vi "KNN clasification.vi"() -> ()   [LabVIEW 2014]
uses:
  <vilib>/Utility/file.llb/Write To Spreadsheet File (string).vi
panel:
  out "results":string[][](array[string])
  in  "cluster centers (original) 2":string[](array[string])=["1 0 -1 1 -1 0 -4 1 -4 0 1", "2 0 -1 2 -1 0 -2 2 -2 0 2", "3 0 -3 3 -3 0 -2 3 -2 0 3", "4 0 -3 4 -3 0 -4 4 -4 0 4", "-1 1 -4 0 -4 4 -3 4 -4 0 -4 1 -1", "-1 2 -2 0 -2 3 -3 3 -2 0 -2 2 -1", "-4 1 -1 0 -1 2 -2 2 -1 0 -1 1 -4", "-4 4 -3 0 -3 3 -2 3 -3 0 -3 4 -4", "0 -4 1 -1 0 -3 3 -2 3 -3 0 -1 1 -4 0", "0 -4 4 -3 0 -1 2 -2 2 -1 0 -3 4 -4 0"]
  in  "cluster centers 2 centers for diagonals - short - original clusters":string[](array[string])=["1 0 -1 1 -1 0 -4 1 -4 0 1", "2 0 -1 2 -1 0 -2 2 -2 0 2", "3 0 -3 3 -3 0 -2 3 -2 0 3", "4 0 -3 4 -3 0 -4 4 -4 0 4", "-1 1 -4 0 -4 4 -3 4 -4 0 -4 1 -1", "-1 2 -2 0 -2 3 -3 3 -2 0 -2 2 -1", "-4 1 -1 0 -1 2 -2 2 -1 0 -1 1 -4", "-4 4 -3 0 -3 3 -2 3 -3 0 -3 4 -4", "0 1 -1 0 -3 3 0 3 -3 0 -1 1 0", "0 1 -4 0 -2 3 0 3 -2 0 -4 1 0", "0 4 -3 0 -1 2 0 2 -1 0 -3 4 0", "0 4 -4 0 -2 2 0 2 -2 0 -4 4 0"]
  in  "cluster centers (original)":string[](array[string])=["1 0 -1 1 -1 0 -4 1 -4 0 1", "2 0 -1 2 -1 0 -2 2 -2 0 2", "3 0 -3 3 -3 0 -2 3 -2 0 3", "4 0 -3 4 -3 0 -4 4 -4 0 4", "-1 1 -4 0 -4 4 -3 4 -4 0 -4 1 -1", "-1 2 -2 0 -2 3 -3 3 -2 0 -2 2 -1", "-4 1 -1 0 -1 2 -2 2 -1 0 -1 1 -4", "-4 4 -3 0 -3 3 -2 3 -3 0 -3 4 -4", "0 -4 1 -1 0 -3 3 -2 3 -3 0 -1 1 -4 0", "0 -4 4 -3 0 -1 2 -2 2 -1 0 -3 4 -4 0"]
  out "data to save":string[][](array[string])
  out "position only":string[][](array[string])
  out "non directional transition":string[][](array[string])
  in  "ALL data in checked":string[][](array[string])=array2194x3[6582 elements]
  in  "from CSS validation cluster centers 2 centers for diagonals - long - original clusters 3":string[](array[string])=["1 0 -1 1 -1 0 -4 1 -4 0 1 0 -1 1 -1 0 -4 1 -4 0 1 0 -1 1 -1 0 -4 1 -4 0 1", "2 0 -1 2 -1 0 -2 2 -2 0 2 0 -1 2 -1 0 -2 2 -2 0 2 0 -1 2 -1 0 -2 2 -2 0 2", "3 0 -3 3 -3 0 -2 3 -2 0 3 0 -3 3 -3 0 -2 3 -2 0 3 0 -3 3 -3 0 -2 3 -2 0 3", "4 0 -3 4 -3 0 -4 4 -4 0 4 0 -3 4 -3 0 -4 4 -4 0 4 0 -3 4 -3 0 -4 4 -4 0 4", "-1 1 -4 0 -4 4 -3 4 -4 0 -4 1 -1 1 -4 0 -4 4 -3 4 -4 0 -4 1 -1 1 -4 0 -4 4 -3 4 -4 0 -4 1 -1", "-1 2 -2 0 -2 3 -3 3 -2 0 -2 2 -1 2 -2 0 -2 3 -3 3 -2 0 -2 2 -1 2 -2 0 -2 3 -3 3 -2 0 -2 2 -1", "-4 1 -1 0 -1 2 -2 2 -1 0 -1 1 -4 1 -1 0 -1 2 -2 2 -1 0 -1 1 -4 1 -1 0 -1 2 -2 2 -1 0 -1 1 -4", "-4 4 -3 0 -3 3 -2 3 -3 0 -3 4 -4 4 -3 0 -3 3 -2 3 -3 0 -3 4 -4 4 -3 0 -3 3 -2 3 -3 0 -3 4 -4", "0 1 -1 0 -3 3 0 3 -3 0 -1 1 0 1 -1 0 -3 3 0 3 -3 0 -1 1 0 1 -1 0 -3 3 0 3 -3 0 -1 1 0 ", "0 1 -4 0 -2 3 0 3 -2 0 -4 1 0 1 -4 0 -2 3 0 3 -2 0 -4 1 0 1 -4 0 -2 3 0 3 -2 0 -4 1 0", "0 4 -3 0 -1 2 0 2 -1 0 -3 4 0 4 -3 0 -1 2 0 2 -1 0 -3 4 0 4 -3 0 -1 2 0 2 -1 0 -3 4 0", "0 4 -4 0 -2 2 0 2 -2 0 -4 4 0 4 -4 0 -2 2 0 2 -2 0 -4 4 0 4 -4 0 -2 2 0 2 -2 0 -4 4 0"]
  out "output 2":string[][](array[string])
  in  "K":i32
  in  "cluster centers 2 centers for diagonals - short clusters  with zero side clusters 3 (mod)":string[](array[string])=["0 1 0 -1 1 0 1 -1 0 -4 1 0 1 -4 0", "0 2 0 -1 2 0 2 -1 0 -2 2 0 2 -2 0", "0 3 0 -3 3 0 3 -3 0 -2 3 0 3 -2 0", "0 4 0 -3 4 0 4 -3 0 -4 4 0 4 -4 0", "0 1 0 1 -4 0 -4 4 0 4 0 4 0 4 -4 0 -4 1 0 1 0", "0 2 0 2 -2 0 -2 3 0 3 0 3 0 3 -2 0 -2 2 0 2 0", "0 1 0 1 -1 0 -1 2 0 2 0 2 0 2 -1 0 -1 1 0 1 0", "0 4 0 4 -3 0 -3 3 0 3 0 3 0 3 -3 0 -3 4 0 4 0", "0 1 -1 0 -3 3 0 3 -3 0 -1 1 0 1 -1 0 -3 3 0 3 -3 0 -1 1 0", "0 1 -4 0 -2 3 0 3 -2 0 -4 1 0 1 -4 0 -2 3 0 3 -2 0 -4 1 0", "0 4 -3 0 -1 2 0 2 -1 0 -3 4 0 4 -3 0 -1 2 0 2 -1 0 -3 4 0", "0 4 -4 0 -2 2 0 2 -2 0 -4 4 0 4 -4 0 -2 2 0 2 -2 0 -4 4 0"]
  in  "cluster centers 2 centers for diagonals - short clusters  with zero side clusters 2":string[](array[string])=["0 1 0 -1 1 0 1 -1 0 -4 1 0 1 -4 0", "0 2 0 -1 2 0 2 -1 0 -2 2 0 2 -2 0", "0 3 0 -3 3 0 3 -3 0 -2 3 0 3 -2 0", "0 4 0 -3 4 0 4 -3 0 -4 4 0 4 -4 0", "0 -1 1 0 1 -4 0 -4 4 0 4 -3 0 -3 4 0 4 -4 0 -4 1 0 1 -1 0", "0 -1 2 0 2 -2 0 -2 3 0 3 -3 0 -3 3 0 3 -2 0 -2 2 0 2 -1 0", "0 -4 1 0 1 -1 0 -1 2 0 2 -2 0 -2 2 0 2 -1 0 -1 1 0 1 -4 0", "0 -4 4 0 4 -3 0 -3 3 0 3 -2 0 -2 3 0 3 -3 0 -3 4 0 4 -4 0", "0 1 -1 0 -3 3 0 3 -3 0 -1 1 0 1 -1 0 -3 3 0 3 -3 0 -1 1 0", "0 1 -4 0 -2 3 0 3 -2 0 -4 1 0 1 -4 0 -2 3 0 3 -2 0 -4 1 0", "0 4 -3 0 -1 2 0 2 -1 0 -3 4 0 4 -3 0 -1 2 0 2 -1 0 -3 4 0", "0 4 -4 0 -2 2 0 2 -2 0 -4 4 0 4 -4 0 -2 2 0 2 -2 0 -4 4 0"]
  in  "cluster centers 2 centers for diagonals - long clusters  with zero side clusters":string[](array[string])=["0 1 0 -1 1 0 1 -1 0 -4 1 0 1 -4 0 1 0 -1 1 0 1 -1 0 -4 1 0 1 -4 0", "0 2 0 -1 2 0 2 -1 0 -2 2 0 2 -2 0 2 0 -1 2 0 2 -1 0 -2 2 0 2 -2 0", "0 3 0 -3 3 0 3 -3 0 -2 3 0 3 -2 0 3 0 -3 3 0 3 -3 0 -2 3 0 3 -2 0", "0 4 0 -3 4 0 4 -3 0 -4 4 0 4 -4 0 4 0 -3 4 0 4 -3 0 -4 4 0 4 -4 0", "0 -1 1 -4 0 -4 4 -3 0 -3 4 -4 0 -4 1 -1 0 -1 1 -4 0 -4 4 -3 0 -3 4 -4 0 -4 1 -1 0", "0 -1 2 -2 0 -2 3 -3 0 -3 3 -2 0 -2 2 -1 0 -1 2 -2 0 -2 3 -3 0 -3 3 -2 0 -2 2 -1 0", "0 -4 1 -1 0 -1 2 -2 0 -2 2 -1 0 -1 1 -4 0 -4 1 -1 0 -1 2 -2 0 -2 2 -1 0 -1 1 -4 0", "0 -4 4 -3 0 -3 3 -2 0 -2 3 -3 0 -3 4 -4 0 -4 4 -3 0 -3 3 -2 0 -2 3 -3 0 -3 4 -4 0", "0 1 -1 0 -3 3 0 3 -3 0 -1 1 0 1 -1 0 -3 3 0 3 -3 0 -1 1 0", "0 1 -4 0 -2 3 0 3 -2 0 -4 1 0 1 -4 0 -2 3 0 3 -2 0 -4 1 0", "0 4 -3 0 -1 2 0 2 -1 0 -3 4 0 4 -3 0 -1 2 0 2 -1 0 -3 4 0", "0 4 -4 0 -2 2 0 2 -2 0 -4 4 0 4 -4 0 -2 2 0 2 -2 0 -4 4 0", ""]
  in  "cluster centers 2 long":string[](array[string])=["0 1 0 -1 1 0 1 -1 0 -4 1 0 1 -4 0 1 0 -1 1 0 1 -1 0 -4 1 0 1 -4 0", "0 2 0 -1 2 0 2 -1 0 -2 2 0 2 -2 0 2 0 -1 2 0 2 -1 0 -2 2 0 2 -2 0", "0 3 0 -3 3 0 3 -3 0 -2 3 0 3 -2 0 3 0 -3 3 0 3 -3 0 -2 3 0 3 -2 0", "0 4 0 -3 4 0 4 -3 0 -4 4 0 4 -4 0 4 0 -3 4 0 4 -3 0 -4 4 0 4 -4 0", "0 -1 1 -4 0 -4 4 -3 4 -4 0 -4 1 -1 0 -1 1 -4 0 -4 4 -3 4 -4 0 -4 1 -1 0", "0 -1 2 -2 0 -2 3 -3 3 -2 0 -2 2 -1 0 -1 2 -2 0 -2 3 -3 3 -2 0 -2 2 -1 0", "0 -4 1 -1 0 -1 2 -2 2 -1 0 -1 1 -4 0 -4 1 -1 0 -1 2 -2 2 -1 0 -1 1 -4 0", "0 -4 4 -3 0 -3 3 -2 3 -3 0 -3 4 -4 0 -4 4 -3 0 -3 3 -2 3 -3 0 -3 4 -4 0", "0 -4 1 -1 0 -3 3 -2 3 -3 0 -1 1 -4 0 -4 1 -1 0 -3 3 -2 3 -3 0 -1 1 -4 0", "0 -4 4 -3 0 -1 2 -2 2 -1 0 -3 4 -4 0 -4 4 -3 0 -1 2 -2 2 -1 0 -3 4 -4 0"]
  out "directional transitions":string[][](array[string])
  out "Weighted arrays for movement patterns":dbl[][][](array[numeric])
  out "Weighted arrays of cluster centers":dbl[][][](array[numeric])
  in  "Cluster centers":string[](array[string])=["1 0 1 0 1 0 1 0", "2 0 2 0 2 0 2 0", "3 0 3 0 3 0 3 0", "4 0 4 0 4 0 4 0", "1 0 4 0 1 0 4 0", "2 0 3 0 2 0 3 0", "1 0 2 0 1 0 2 0", "3 0 4 0 3 0 4 0", "1 0 3 0 1 0 3 0", "2 0 4 0 2 0 4 0"]
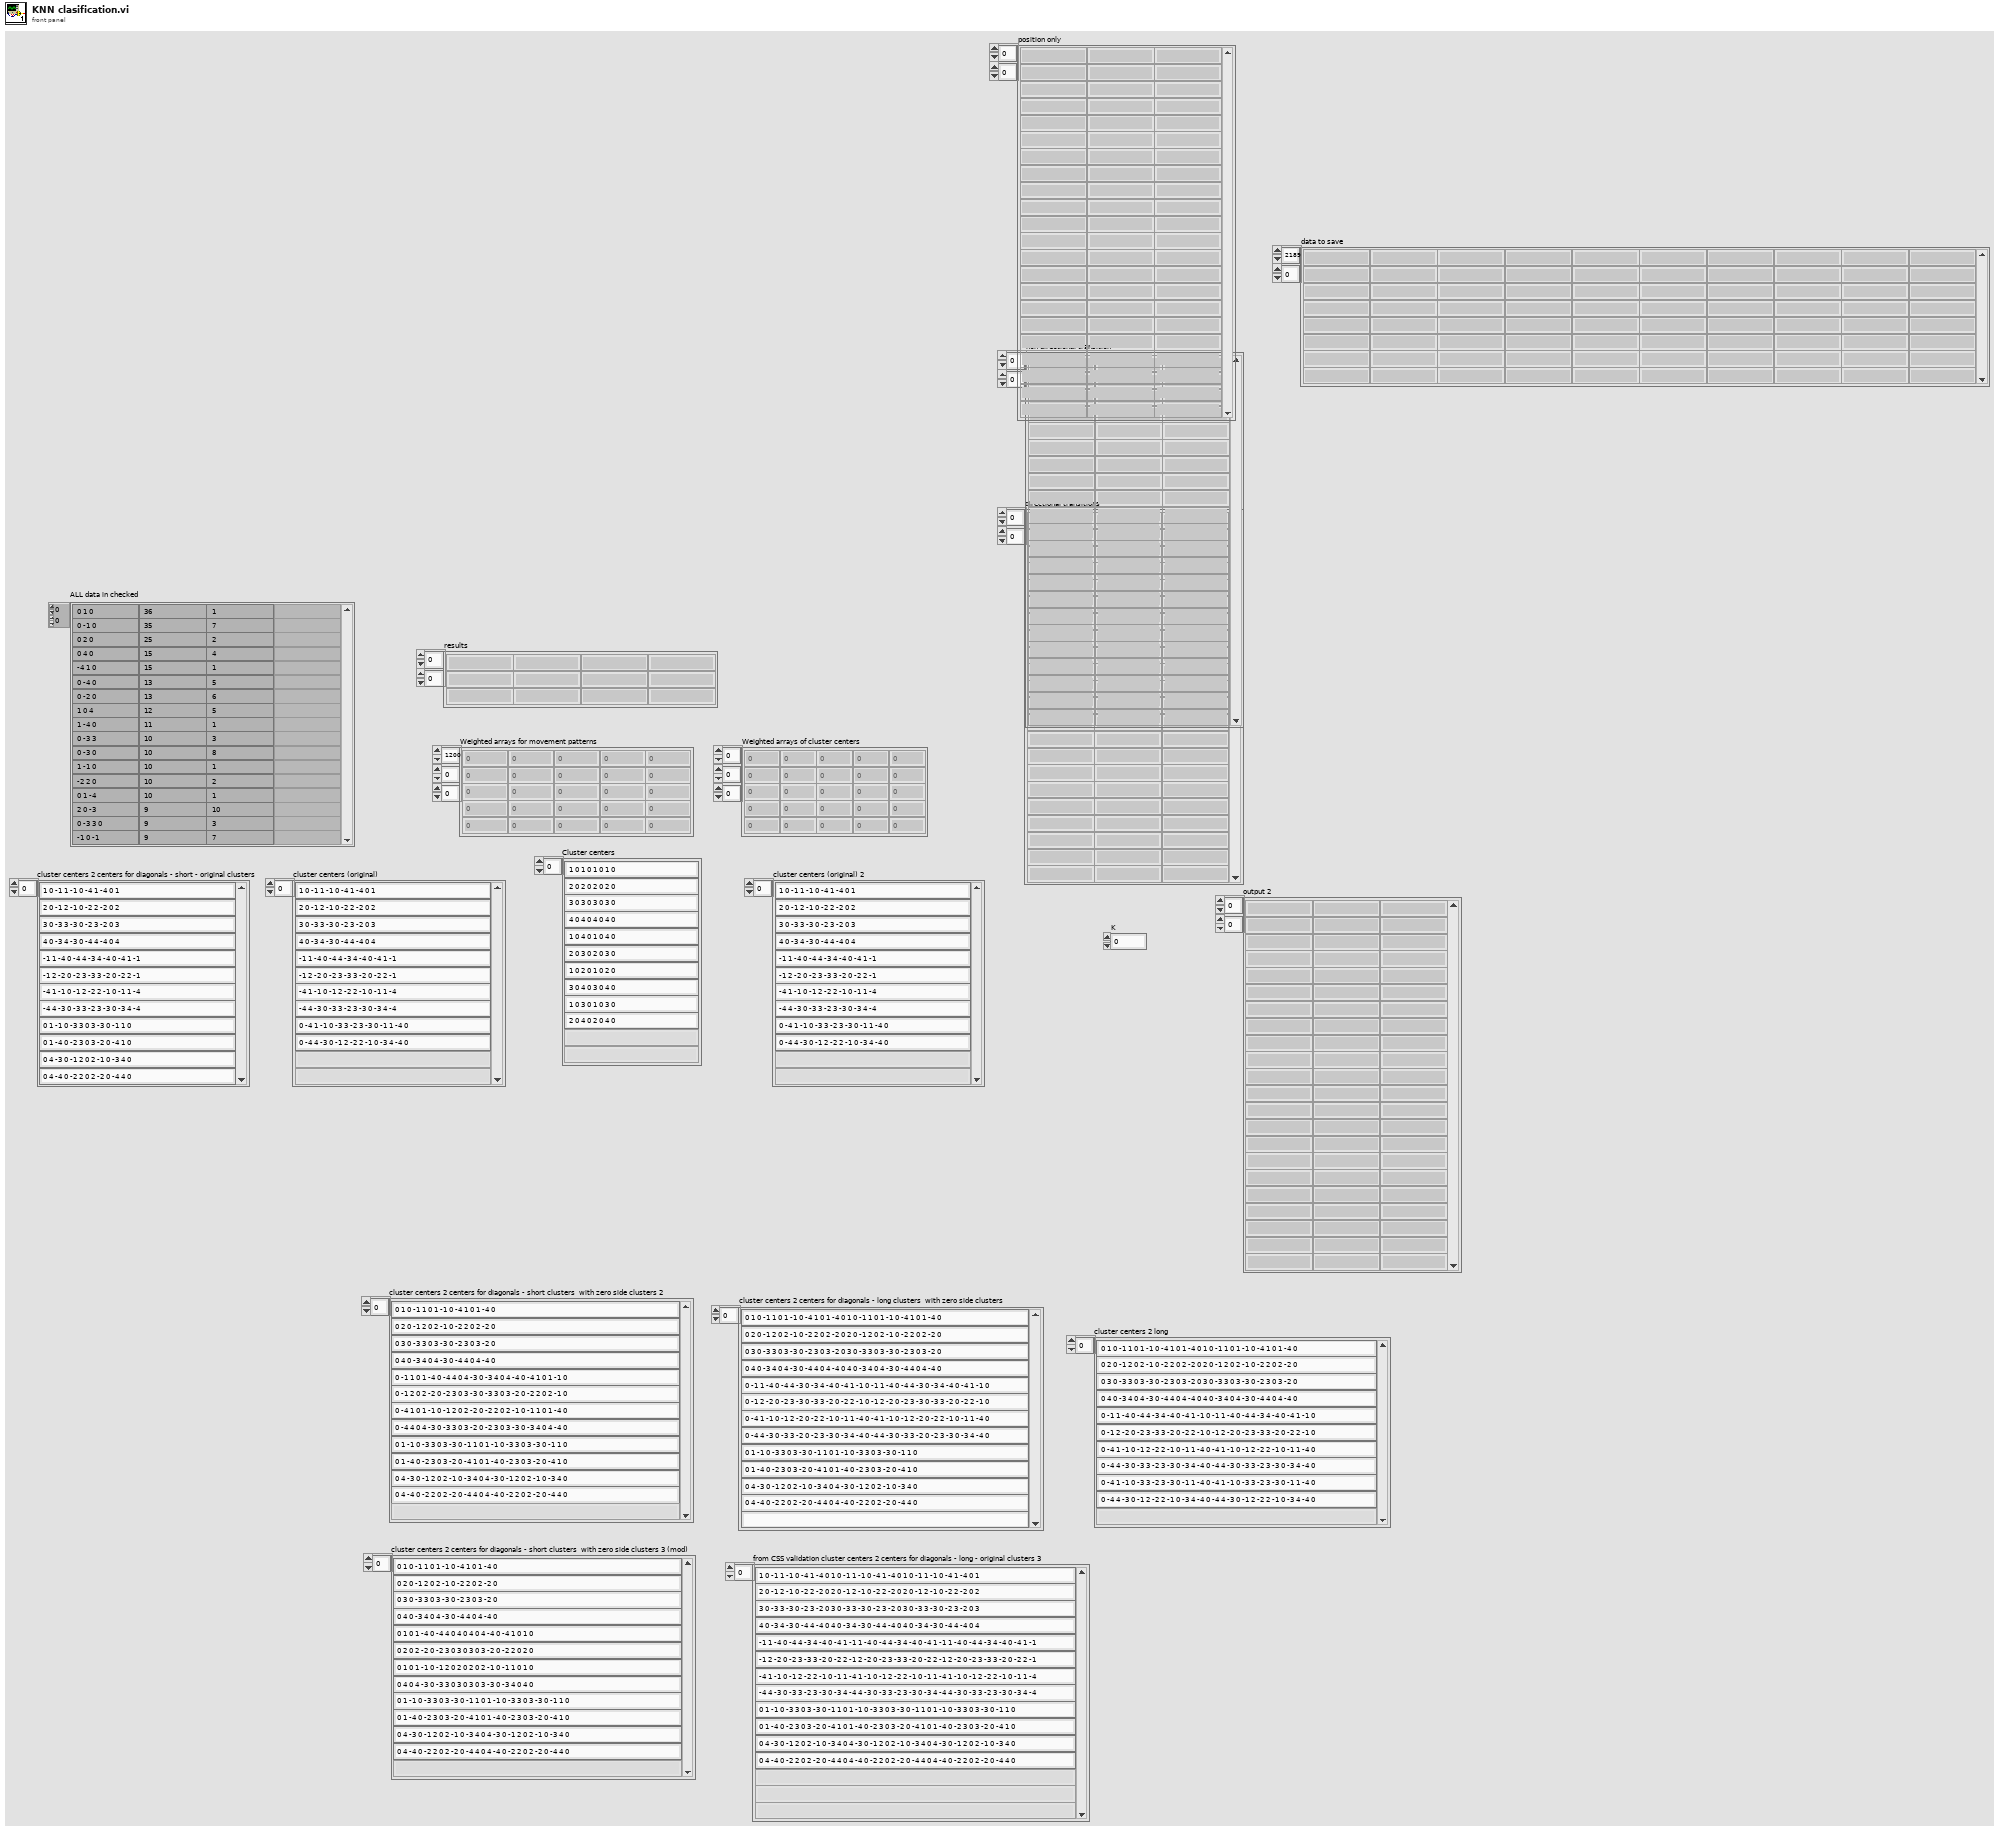
[diagram p1: front panel]
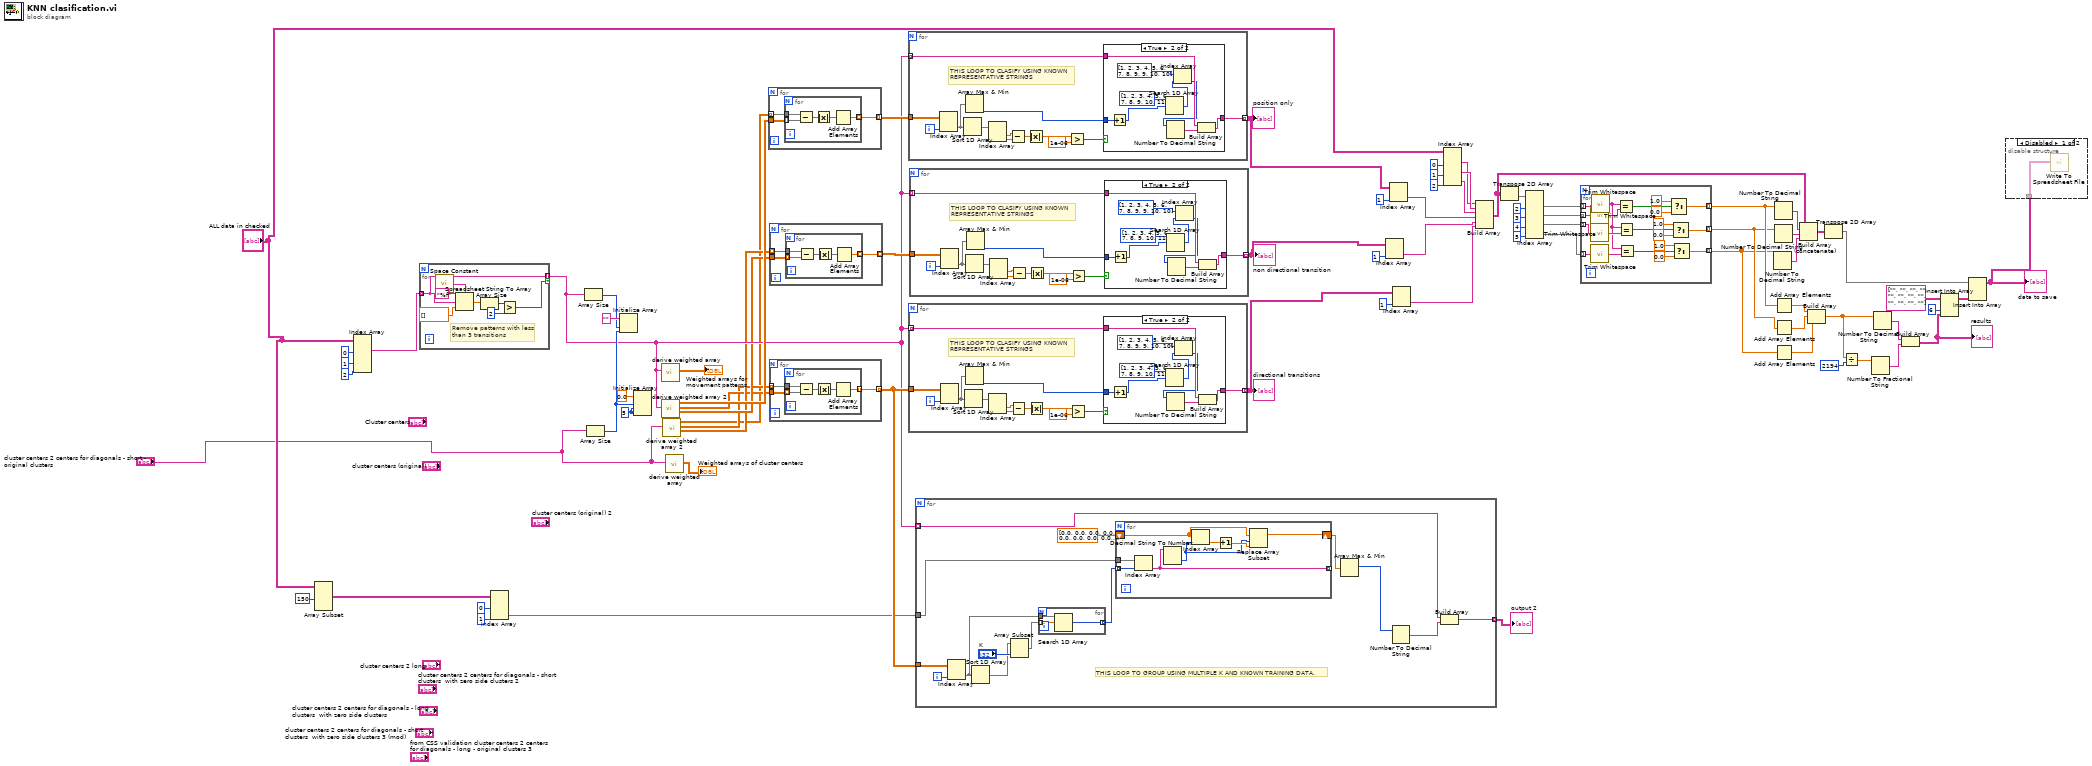
[diagram p0: block diagram]
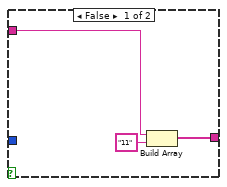
[diagram p3: hidden frame]
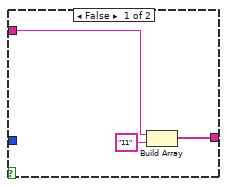
[diagram p4: hidden frame]
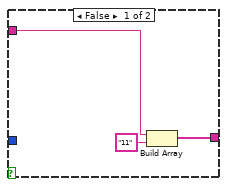
[diagram p5: hidden frame]
diagram:
  w72 = 5 ("dimension size")
  n1 = Array Subset(array="ALL data in checked", length (row)=150 ("length")) -> (w61:string[][])  [unwired: 3 in]
  n2 = Index Array(array="ALL data in checked", index (col) #1=0 ("disabled index (col)"), index (col) #2=1 ("index (col)"), index (col) #3=2 ("index (col)")) -> (element #1=w60:string[])  [unwired: 3 in, 2 out]
  n3 = for {
    tunnel: w60 -> [w77] mode=indexing
    tunnel: [w77] -> w54 mode=indexing if=w76
    # "Remove patterns with less \nthan 3 transitions"
    n4 = call <vilib>:"Space Constant.vi"() -> ("String"=w82:string)
    n5 = Spreadsheet String To Array(delimiter (Tab)=w82, format string="%f", spreadsheet string=w77, array type (2D Dbl)=dbl[] [] ("array 2")) -> (array=w80:dbl[])
    n6 = Array Size(array=w80) -> (size(s)=w79:i32)
    n7 = Greater?(x=w79, y=2) -> (0:w76:bool)
  }
  n8 = Index Array(array=w61, index (col) #1=0 ("disabled index (col)"), index (col) #2=1 ("index (col)")) -> (element #2=w59:string[])  [unwired: 2 in, 1 out]
  n9 = Array Size(array=w54) -> (size(s)=w74:i32)
  n10 = Array Size(array="cluster centers 2 centers for diagonals - short - original clusters") -> (size(s)=w71:i32)
  n11 = Initialize Array("" ("spreadsheet string"), w74, w71) -> ()  [unwired: 1 out]
  n12 = Initialize Array(0.0, w71, w72, w72) -> ()  [unwired: 1 out]
  n13 = call "derive weighted array.vi"("Full transition sequence from service to end"=w54) -> ("Weighted arrays"=→"Weighted arrays for movement patterns":dbl[][][])  [unwired: 10 in]
  n14 = call "derive weighted array 2.vi"("Full transition sequence from service to end"=w54) -> ("weighted array (NON directional transitions)"=w53:dbl[][], "weighted array (directional transitions)"=w51:dbl[][], "weighted array positions only"=w55:dbl[][])  [unwired: 8 in]
  n15 = call "derive weighted array 2.vi"("Full transition sequence from service to end"="cluster centers 2 centers for diagonals - short - original clusters") -> ("weighted array (NON directional transitions)"=w52:dbl[][], "weighted array (directional transitions)"=w50:dbl[][], "weighted array positions only"=w3:dbl[][])  [unwired: 8 in]
  n16 = call "derive weighted array.vi"("Full transition sequence from service to end"="cluster centers 2 centers for diagonals - short - original clusters") -> ("Weighted arrays"=→"Weighted arrays of cluster centers":dbl[][][])  [unwired: 10 in]
  n17 = for {
    tunnel: w3 -> [w86] mode=indexing
    tunnel: w55 -> [w85]
    tunnel: [w84] -> w56 mode=indexing
    n18 = for {
      tunnel: w86 -> [w91]
      tunnel: w85 -> [w90] mode=indexing
      tunnel: [w88] -> w84 mode=indexing
      n19 = Subtract(x=w91, y=w90) -> (x-y=w89:dbl[])
      n20 = Absolute Value(x=w89) -> (abs(x)=w87:dbl[])
      n21 = Add Array Elements(numeric array=w87) -> (sum=w88:dbl)
    }
  }
  n22 = for {
    tunnel: w50 -> [w94] mode=indexing
    tunnel: w51 -> [w93]
    tunnel: [w92] -> w64 mode=indexing
    n23 = for {
      tunnel: w94 -> [w99]
      tunnel: w93 -> [w98] mode=indexing
      tunnel: [w96] -> w92 mode=indexing
      n24 = Subtract(x=w99, y=w98) -> (x-y=w97:dbl[])
      n25 = Absolute Value(x=w97) -> (abs(x)=w95:dbl[])
      n26 = Add Array Elements(numeric array=w95) -> (sum=w96:dbl)
    }
  }
  n27 = for {
    tunnel: w52 -> [w102] mode=indexing
    tunnel: w53 -> [w101]
    tunnel: [w100] -> w57 mode=indexing
    n28 = for {
      tunnel: w102 -> [w107]
      tunnel: w101 -> [w106] mode=indexing
      tunnel: [w104] -> w100 mode=indexing
      n29 = Subtract(x=w107, y=w106) -> (x-y=w105:dbl[])
      n30 = Absolute Value(x=w105) -> (abs(x)=w103:dbl[])
      n31 = Add Array Elements(numeric array=w103) -> (sum=w104:dbl)
    }
  }
  n32 = for {
    tunnel: w54 -> [w110] mode=indexing
    tunnel: w56 -> [w120]
    tunnel: [w108] -> w23 mode=indexing
    i -> [w113]
    # "THIS LOOP TO CLASIFY USING KNOWN \nREPRESENTATIVE STRINGS"
    n33 = Index Array(array=w120, index (col)=w113) -> (element=w112:dbl[])  [unwired: 1 in]
    n34 = Sort 1D Array(array=w112) -> (sorted array=w115:dbl[])
    n35 = Array Max & Min(array=w112) -> (min index (indices)=w111:i32)  [unwired: 3 out]
    n36 = Index Array(array=w115) -> (element #1=w119:dbl, element #2=w114:dbl)  [unwired: 2 in]
    n37 = Subtract(x=w119, y=w114) -> (x-y=w117:dbl)
    n38 = Absolute Value(x=w117) -> (abs(x)=w116:dbl)
    n39 = Greater?(x=w116, y=1e-06) -> (0:w109:bool)
    n40 = case shown="True" w109 {
      tunnel: w111 -> [_ w130]
      tunnel: w110 -> [w122 w129]
      tunnel: [w123 w131] -> w108
      frame False {
        n41 = Build Array(w122, "11" ("element")) -> (w123:string[])
      }
      frame True {
        n42 = Increment(x=w130) -> (x+1=w125:i32)
        n43 = Search 1D Array(1D array=i32[] [1, 2, 3, 4, 5, 6, 7, 8, 9, 10, 11, 12], element=w125) -> (index of element=w128:i32)  [unwired: 1 in]
        n44 = Index Array(array=i32[] [1, 2, 3, 4, 5, 6, 7, 8, 9, 9, 10, 10], index=w128) -> (element=w124:i32)
        n45 = Number To Decimal String(number=w124) -> (decimal integer string=w132:string)  [unwired: 1 in]
        n46 = Build Array(w129, w132) -> (w131:string[])
      }
    }
  }
  "position only" <- w23
  n47 = for {
    tunnel: w54 -> [w135] mode=indexing
    tunnel: w64 -> [w145]
    tunnel: [w133] -> w21 mode=indexing
    i -> [w138]
    # "THIS LOOP TO CLASIFY USING KNOWN \nREPRESENTATIVE STRINGS"
    n48 = Index Array(array=w145, index (col)=w138) -> (element=w137:dbl[])  [unwired: 1 in]
    n49 = Sort 1D Array(array=w137) -> (sorted array=w140:dbl[])
    n50 = Array Max & Min(array=w137) -> (min index (indices)=w136:i32)  [unwired: 3 out]
    n51 = Index Array(array=w140) -> (element #1=w144:dbl, element #2=w139:dbl)  [unwired: 2 in]
    n52 = Subtract(x=w144, y=w139) -> (x-y=w142:dbl)
    n53 = Absolute Value(x=w142) -> (abs(x)=w141:dbl)
    n54 = Greater?(x=w141, y=1e-06) -> (0:w134:bool)
    n55 = case shown="True" w134 {
      tunnel: w136 -> [_ w155]
      tunnel: w135 -> [w147 w154]
      tunnel: [w148 w156] -> w133
      frame False {
        n56 = Build Array(w147, "11" ("element")) -> (w148:string[])
      }
      frame True {
        n57 = Increment(x=w155) -> (x+1=w150:i32)
        n58 = Search 1D Array(1D array=i32[] [1, 2, 3, 4, 5, 6, 7, 8, 9, 10, 11, 12], element=w150) -> (index of element=w153:i32)  [unwired: 1 in]
        n59 = Index Array(array=i32[] [1, 2, 3, 4, 5, 6, 7, 8, 9, 9, 10, 10], index=w153) -> (element=w149:i32)
        n60 = Number To Decimal String(number=w149) -> (decimal integer string=w157:string)  [unwired: 1 in]
        n61 = Build Array(w154, w157) -> (w156:string[])
      }
    }
  }
  "directional transitions" <- w21
  n62 = for {
    tunnel: w54 -> [w160] mode=indexing
    tunnel: w57 -> [w170]
    tunnel: [w158] -> w22 mode=indexing
    i -> [w163]
    # "THIS LOOP TO CLASIFY USING KNOWN \nREPRESENTATIVE STRINGS"
    n63 = Index Array(array=w170, index (col)=w163) -> (element=w162:dbl[])  [unwired: 1 in]
    n64 = Sort 1D Array(array=w162) -> (sorted array=w165:dbl[])
    n65 = Array Max & Min(array=w162) -> (min index (indices)=w161:i32)  [unwired: 3 out]
    n66 = Index Array(array=w165) -> (element #1=w169:dbl, element #2=w164:dbl)  [unwired: 2 in]
    n67 = Subtract(x=w169, y=w164) -> (x-y=w167:dbl)
    n68 = Absolute Value(x=w167) -> (abs(x)=w166:dbl)
    n69 = Greater?(x=w166, y=1e-06) -> (0:w159:bool)
    n70 = case shown="True" w159 {
      tunnel: w161 -> [_ w180]
      tunnel: w160 -> [w172 w179]
      tunnel: [w173 w181] -> w158
      frame False {
        n71 = Build Array(w172, "11" ("element")) -> (w173:string[])
      }
      frame True {
        n72 = Increment(x=w180) -> (x+1=w175:i32)
        n73 = Search 1D Array(1D array=i32[] [1, 2, 3, 4, 5, 6, 7, 8, 9, 10, 11, 12], element=w175) -> (index of element=w178:i32)  [unwired: 1 in]
        n74 = Index Array(array=i32[] [1, 2, 3, 4, 5, 6, 7, 8, 9, 9, 10, 10], index=w178) -> (element=w174:i32)
        n75 = Number To Decimal String(number=w174) -> (decimal integer string=w182:string)  [unwired: 1 in]
        n76 = Build Array(w179, w182) -> (w181:string[])
      }
    }
  }
  "non directional transition" <- w22
  n77 = for {
    tunnel: w64 -> [w196]
    tunnel: w54 -> [w187] mode=indexing
    tunnel: w59 -> [w192]
    tunnel: [w185] -> w63 mode=indexing
    i -> [w195]
    # "THIS LOOP TO GROUP USING MULTIPLE K AND KNOWN TRAINING DATA."
    n78 = Index Array(array=w196, index (col)=w195) -> (element=w183:dbl[])  [unwired: 1 in]
    n79 = Sort 1D Array(array=w183) -> (sorted array=w184:dbl[])
    n80 = Array Subset(array=w184, length="K") -> (w193:dbl[])  [unwired: 1 in]
    n81 = for {
      tunnel: w193 -> [w206] mode=indexing
      tunnel: w183 -> [w207]
      tunnel: [w205] -> w191 mode=indexing
      n82 = Search 1D Array(1D array=w207, element=w206) -> (index of element=w205:i32)  [unwired: 1 in]
    }
    n83 = for {
      tunnel: w192 -> [w204]
      tunnel: w191 -> [w203] mode=indexing
      tunnel: [w202] -> _ mode=indexing
      shift-right: [w197] -> w189
      shift-left: dbl[] [0.0, 0.0, 0.0, 0.0, 0.0, 0.0, 0.0, 0.0, 0.0, 0.0, 0.0, 0.0] -> [w200]
      n84 = Index Array(array=w204, index=w203) -> (element=w202:string)
      n85 = Decimal String To Number(string=w202) -> (number=w198:i32)  [unwired: 2 in, 1 out]
      n86 = Index Array(array=w200, index=w198) -> (element=w201:dbl)
      n87 = Increment(x=w201) -> (x+1=w199:dbl)
      n88 = Replace Array Subset(array=w200, new element=w199, index=w198) -> (w197:dbl[])
    }
    n89 = Array Max & Min(array=w189) -> (max index (indices)=w188:i32)  [unwired: 3 out]
    n90 = Number To Decimal String(number=w188) -> (decimal integer string=w186:string)  [unwired: 1 in]
    n91 = Build Array(w187, w186) -> (w185:string[])
  }
  "output 2" <- w63
  n92 = Index Array(array=w22, index (col)=1 ("disabled index (col)")) -> (element=w48:string[])  [unwired: 1 in]
  n93 = Index Array(array=w23, index (col)=1 ("disabled index (col)")) -> (element=w47:string[])  [unwired: 1 in]
  n94 = Index Array(array=w21, index (col)=1 ("disabled index (col)")) -> (element=w49:string[])  [unwired: 1 in]
  n95 = Index Array(array="ALL data in checked", index (col) #1=0 ("disabled index (col)"), index (col) #2=1 ("index (col)"), index (col) #3=2 ("index (col)")) -> (element #1=w24:string[], element #2=w45:string[], element #3=w46:string[])  [unwired: 3 in]
  n96 = Build Array(w24, w45, w46, w47, w48, w49) -> (w35:string[][])
  n97 = Transpose 2D Array(2D array=w35) -> (transposed array=w32:string[][])
  n98 = Index Array(array=w32, index (col) #1=2 ("disabled index (col)"), index (col) #2=3 ("index (col)"), index (col) #3=4 ("index (col)"), index (col) #4=5 ("index (col)")) -> (element #1=w29:string[], element #2=w30:string[], element #3=w31:string[], element #4=w38:string[])  [unwired: 4 in]
  n99 = for {
    tunnel: w29 -> [w219] mode=indexing
    tunnel: w30 -> [w218] mode=indexing
    tunnel: w31 -> [w217] mode=indexing
    tunnel: [w221] -> w19 mode=indexing
    tunnel: [w220] -> w18 mode=indexing
    tunnel: w38 -> [w212] mode=indexing
    tunnel: [w208] -> w17 mode=indexing
    n100 = call <vilib>:"Trim Whitespace.vi"("string"=w218) -> ("trimmed string"=w216:string)  [unwired: 1 in]
    n101 = call <vilib>:"Trim Whitespace.vi"("string"=w217) -> ("trimmed string"=w215:string)  [unwired: 1 in]
    n102 = call <vilib>:"Trim Whitespace.vi"("string"=w212) -> ("trimmed string"=w214:string)  [unwired: 1 in]
    n103 = call <vilib>:"Trim Whitespace.vi"("string"=w219) -> ("trimmed string"=w213:string)  [unwired: 1 in]
    n104 = Equal?(x=w213, y=w216) -> (x = y?=w227:bool)
    n105 = Equal?(x=w213, y=w215) -> (x = y?=w222:bool)
    n106 = Equal?(x=w213, y=w214) -> (x = y?=w209:bool)
    n107 = Select(t=1.0, s=w227, f=0.0) -> (s? t:f=w221:dbl)
    n108 = Select(t=1.0, s=w222, f=0.0) -> (s? t:f=w220:dbl)
    n109 = Select(t=1.0, s=w209, f=0.0) -> (s? t:f=w208:dbl)
  }
  n110 = Number To Decimal String(number=w17) -> (decimal integer string=w39:string[])  [unwired: 1 in]
  n111 = Number To Decimal String(number=w19) -> (decimal integer string=w33:string[])  [unwired: 1 in]
  n112 = Number To Decimal String(number=w18) -> (decimal integer string=w34:string[])  [unwired: 1 in]
  n113 = Add Array Elements(numeric array=w17) -> (sum=w14:dbl)
  n114 = Add Array Elements(numeric array=w19) -> (sum=w16:dbl)
  n115 = Add Array Elements(numeric array=w18) -> (sum=w15:dbl)
  n116 = Build Array (concatenate)(w35, w33, w34, w39) -> (w36:string[][])
  n117 = Build Array(w16, w15, w14) -> (w12:dbl[])
  n118 = Transpose 2D Array(2D array=w36) -> (transposed array=w4:string[][])
  n119 = Divide(x=w12, y=2194 ("f")) -> (x/y=w11:dbl[])
  n120 = Number To Fractional String(number=w11) -> (F-format string=w9:string[])  [unwired: 3 in]
  n121 = Number To Decimal String(number=w12) -> (decimal integer string=w10:string[])  [unwired: 1 in]
  n122 = Build Array(w10, w9) -> (w2:string[][])
  "results" <- w2
  n123 = Insert Into Array(array=string[][] [["", "", "", "", "", ""], ["", "", "", "", "", ""]] ("appended array 3"), index (col)=6 ("disabled index (col)"), new element=w2) -> (w5:string[][])  [unwired: 1 in]
  n124 = Insert Into Array(array=w4, new element=w5) -> (w6:string[][])  [unwired: 2 in]
  "data to save" <- w6
  n125 = disable-structure shown="Disabled" {
    disable-tunnel: w6 -> [w228 _]
    frame Disabled {
      n126 = call-poly <vilib>:"Write To Spreadsheet File.vi"("2D data"=w228) -> ()  [unwired: 7 in, 1 out]
    }
    frame Enabled {
    }
  }
